vi "pid yaw.vi"(6 "yaw":dbl(knob) scale=-180.0..180.0, 8 "spin":dbl(slide) scale=-1.0..1.0, 10 "x":dbl(slide) scale=-1.0..1.0, 11 "y":dbl(slide) scale=-1.0..1.0) -> (3 "yaw setpoint":dbl(knob) scale=0.0..360.0)   [LabVIEW 2023]
uses:
  <vilib>/addons/control/pid/pid.llb/PID (DBL).vi
  <vilib>/addons/control/pid/NI_PID_pid.lvlib
panel:
  in  "PID gains":T1={"proportional gain (Kc)"=1.0, "integral time (Ti, min)"=0.01, "derivative time (Td, min)"=0.0} {"derivative time (Td, min)" format="%.3f"; "integral time (Ti, min)" format="%.3f"; "proportional gain (Kc)" format="%.3f"}
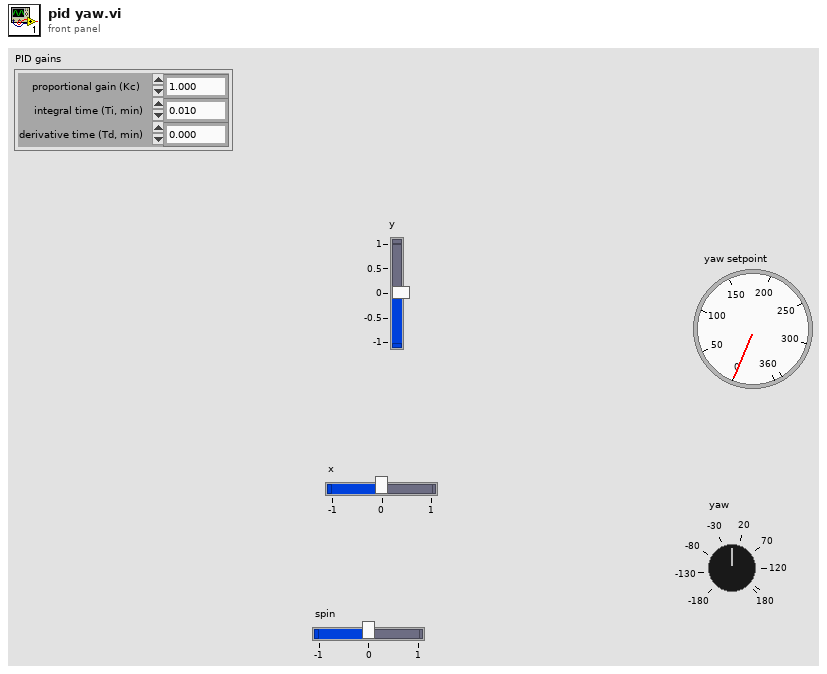
[diagram p1: front panel]
types:
  T1 = cluster{"proportional gain (Kc)":dbl, "integral time (Ti, min)":dbl, "derivative time (Td, min)":dbl}
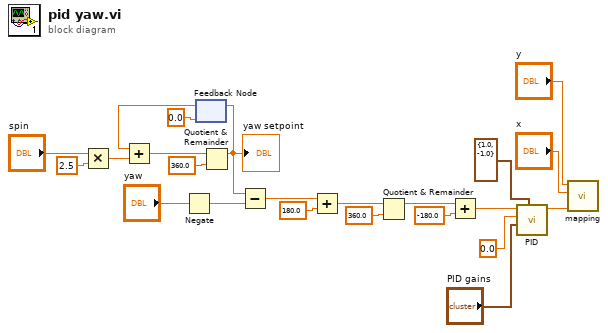
[diagram p0: block diagram]
diagram:
  n1 = Multiply(x="spin", y=2.5) -> (x*y=w19:dbl)
  n2 = Negate(x="yaw") -> (-x=w1:dbl)
  n3 = feedback #1(0.0) -> (w20:dbl)
  n4 = Add(x=w20, y=w19) -> (x+y=w16:dbl)
  n5 = Quotient & Remainder(x=w16, y=360.0) -> (x-y*floor(x/y)=w14:dbl)  [unwired: 1 out]
  "yaw setpoint" <- w14
  n6 = feedback-in #1(w14) -> ()
  n7 = Subtract(x=w14, y=w1) -> (x-y=w13:dbl)
  n8 = Add(x=w13, y=180.0) -> (x+y=w11:dbl)
  n9 = Quotient & Remainder(x=w11, y=360.0) -> (x-y*floor(x/y)=w8:dbl)  [unwired: 1 out]
  n10 = Add(x=w8, y=-180.0) -> (x+y=w7:dbl)
  n11 = call-poly <vilib>:"PID.vi"("output range"=cluster{"output high":dbl, "output low":dbl} {"output high"=1.0, "output low"=-1.0}, "PID gains"="PID gains", "process variable"=0.0, "setpoint"=w7) -> ("output"=w3:dbl)  [unwired: 6 in, 1 out]
  n12 = call "mapping.vi"("spin"=w3, "x"="x", "y"="y") -> ()  [unwired: 9 in]
